vi "Fft.vi"(6 "Chirp Parameters (in)":T1, 8 "error in (no error)":errorcluster, 9 "NumDataPoints":u32, 10 "ChirpedData in":csg[](array[numeric]), 11 "SETI_LV_FPGA in":refnum<class "SETI_LV_FPGA.lvclass">) -> (0 "error out":errorcluster, 1 "NumDataPoints":u32, 2 "FftData out":csg[](array[numeric]), 3 "SETI_LV_FPGA out":refnum<class "SETI_LV_FPGA.lvclass">)   [LabVIEW 2015, in "SETI_LV_FPGA.lvclass"]
uses:
  SETI_LV_FPGA.lvclass
  SETI_LV/TypeDefs/ChirpFFT Pairs.ctl
  SETI_LV/SETI_LV.lvlib
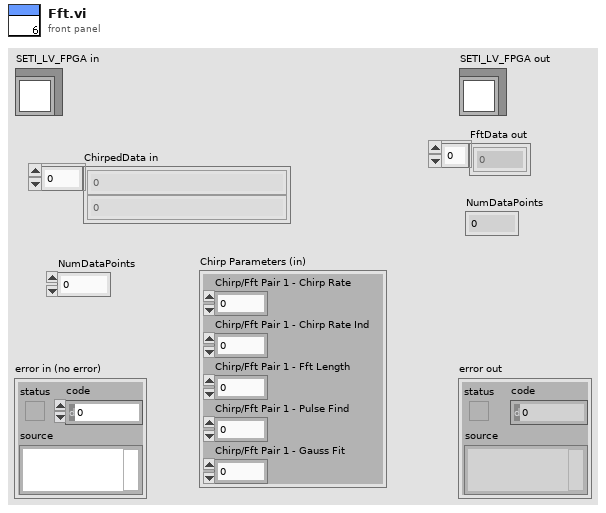
[diagram p1: front panel]
types:
  T1 = typedef "SETI_LV.lvlib/ChirpFFT Pairs.ctl" = cluster{"Chirp/Fft Pair 1 - Chirp Rate":dbl, "Chirp/Fft Pair 1 - Chirp Rate Ind":i32, "Chirp/Fft Pair 1 - Fft Length":i32, "Chirp/Fft Pair 1 - Pulse Find":i32, "Chirp/Fft Pair 1 - Gauss Fit":i32}
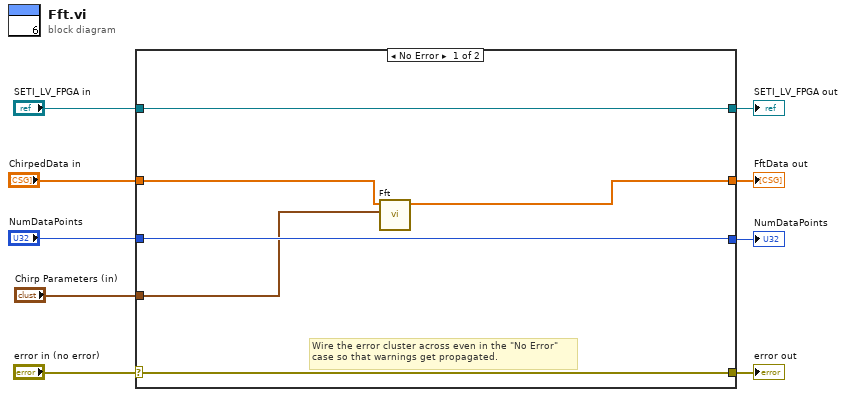
[diagram p0: block diagram]
diagram:
  n1 = case shown="No Error" "error in (no error)" {
    selector: "error in (no error)" -> [w14 w19]
    tunnel: [w14 w19] -> w8
    tunnel: [w15 w18] -> w6
    tunnel: "SETI_LV_FPGA in" -> [w15 w18]
    tunnel: "ChirpedData in" -> [w12 w17]
    tunnel: [w13 w16] -> w2
    tunnel: "NumDataPoints" -> [w13 w16]
    tunnel: [w10 w17] -> w3
    tunnel: "Chirp Parameters (in)" -> [w11 _]
    frame No Error {
      # "Wire the error cluster across even in the \"No Error\"\ncase so that warnings get propagated."
      n2 = call "Fft.vi"("Chirp Parameters (in)"=w11, "DataPoints (in)"=w12) -> ("Fft Results (out)"=w10:csg[])  [unwired: 9 in]
    }
    frame Error {
    }
  }
  "error out" <- w8
  "SETI_LV_FPGA out" <- w6
  "FftData out" <- w3
  "NumDataPoints" <- w2
